vi "Day 7.1 - .vi"(11 "input":string[](array[string])) -> (1 "Sizes":i32[](array[numeric]), 2 "Dirs":string[](array[string]), 3 "output":u64)   [LabVIEW 2021]
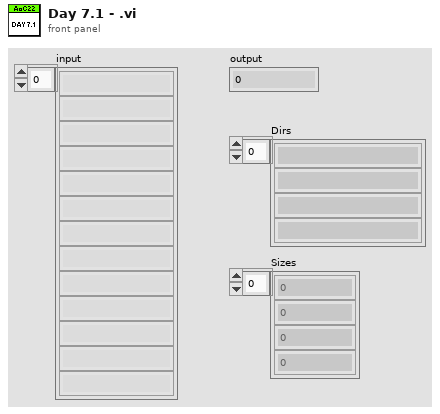
[diagram p1: front panel]
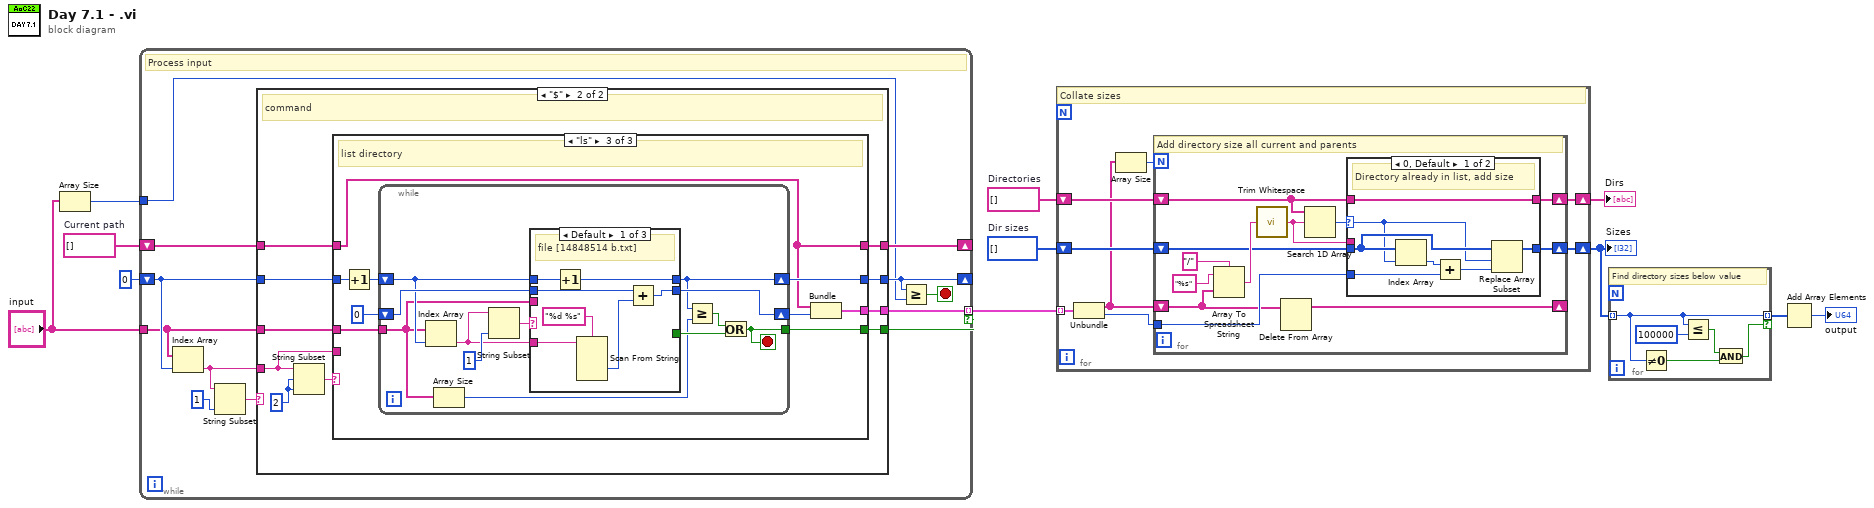
[diagram p0: block diagram]
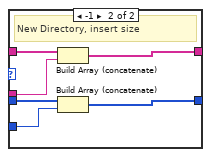
[diagram p2: hidden frame]
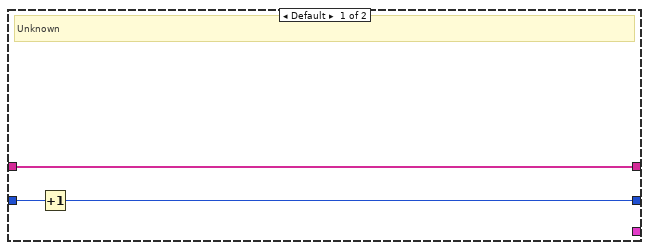
[diagram p3: hidden frame]
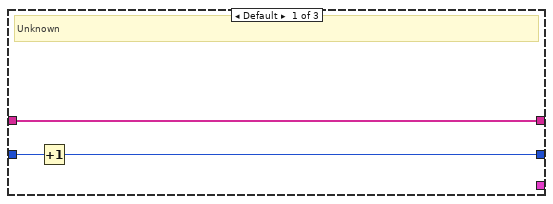
[diagram p4: hidden frame]
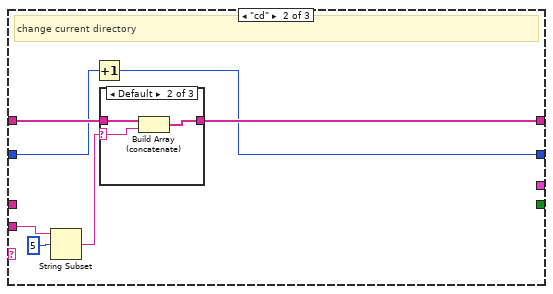
[diagram p5: hidden frame]
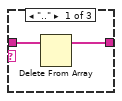
[diagram p6: hidden frame]
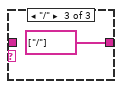
[diagram p7: hidden frame]
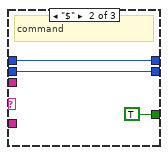
[diagram p8: hidden frame]
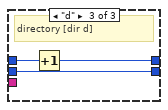
[diagram p9: hidden frame]
diagram:
  w3 = i32[] []  # Dir sizes
  w6 = string[] []  # Directories
  w10 = string[] []  # Current path
  n1 = Array Size(array="input") -> (size(s)=w8:i32)
  n2 = while {
    tunnel: "input" -> [w14]
    shift-right: [w17] -> _
    shift-left: i16 0 -> [w18]
    shift-right: [w20] -> _
    shift-left: w10 -> [w21]
    tunnel: w8 -> [w16]
    tunnel: [w13] -> w4 mode=indexing if=w12
    stop <- w15 stop-if-true
    # "Process input"
    n3 = Index Array(array=w14, index=w18) -> (element=w19:string)
    n4 = String Subset(string=w19, length (rest)=1 ("length (rest)")) -> (substring=w22:string)  [unwired: 1 in]
    n5 = case shown="\"$\"" w22 {
      tunnel: w19 -> [_ w35]
      tunnel: w21 -> [w26 w34]
      tunnel: [w26 w33] -> w20
      tunnel: w18 -> [w25 w32]
      tunnel: [w24 w31] -> w17
      tunnel: w14 -> [_ w30]
      tunnel: [_ w29] -> w13
      tunnel: [_ w28] -> w12
      frame Default {
        # "Unknown"
        n6 = Increment(x=w25) -> (x+1=w24:i16)
      }
      frame "$" {
        w27 = 2 ("length (rest)")
        # "command"
        n7 = String Subset(string=w35, offset (0)=w27, length (rest)=w27) -> (substring=w36:string)
        n8 = case shown="\"ls\"" w36 {
          tunnel: w35 -> [_ w46 _]
          tunnel: w34 -> [w39 w43 w53]
          tunnel: [w39 w42 w53] -> w33
          tunnel: w32 -> [w38 w41 w61]
          tunnel: [w37 w40 w58] -> w31
          tunnel: w30 -> [_ _ w60]
          tunnel: [_ _ w55] -> w29
          tunnel: [_ _ w54] -> w28
          frame Default {
            # "Unknown"
            n9 = Increment(x=w38) -> (x+1=w37:i16)
          }
          frame "cd" {
            # "change current directory"
            n10 = String Subset(string=w46, offset (0)=5) -> (substring=w44:string)  [unwired: 1 in]
            n11 = Increment(x=w41) -> (x+1=w40:i16)
            n12 = case shown="Default" w44 {
              selector: w44 -> [_ w50 _]
              tunnel: w43 -> [w48 w51 _]
              tunnel: [w47 w49 string[] ["/"]] -> w42
              frame ".." {
                n13 = Delete From Array(array=w48) -> (array with subset deleted=w47:string[])  [unwired: 2 in, 1 out]
              }
              frame Default {
                n14 = Build Array (concatenate)(w51, w50) -> (w49:string[])
              }
              frame "/" {
              }
            }
          }
          frame "ls" {
            # "list directory"
            n15 = Increment(x=w61) -> (x+1=w59:i16)
            n16 = while {
              tunnel: w60 -> [w65]
              shift-right: [w66] -> w58
              shift-left: w59 -> [w68]
              shift-right: [w70] -> w56
              shift-left: 0 -> [w71]
              tunnel: [w63] -> w54
              stop <- w63 stop-if-true
              n17 = Index Array(array=w65, index=w68) -> (element=w67:string)
              n18 = Array Size(array=w65) -> (size(s)=w64:i32)
              n19 = String Subset(string=w67, length (rest)=1 ("length (rest)")) -> (substring=w72:string)  [unwired: 1 in]
              n20 = case shown="Default" w72 {
                tunnel: w65 -> [_ _ _]
                tunnel: w68 -> [w80 w82 w86]
                tunnel: [w74 w82 w85] -> w66
                tunnel: [_ TRUE _] -> w69
                tunnel: w67 -> [w79 _ _]
                tunnel: w71 -> [w77 w81 w84]
                tunnel: [w75 w81 w84] -> w70
                frame Default {
                  # "file [14848514 b.txt]"
                  n21 = Increment(x=w80) -> (x+1=w74:i16)
                  n22 = Scan From String(format string="%d %s", input string=w79) -> (output 1=w76:i32)  [unwired: 5 in, 3 out]
                  n23 = Add(x=w77, y=w76) -> (x+y=w75:i32)
                }
                frame "$" {
                  # "command"
                }
                frame "d" {
                  # "directory [dir d]"
                  n24 = Increment(x=w86) -> (x+1=w85:i16)
                }
              }
              n25 = Greater Or Equal?(x=w66, y=w64) -> (x >= y?=w62:bool)
              n26 = Or(x=w62, y=w69) -> (x .or. y?=w63:bool)
            }
            n27 = Bundle("Current path"=w53, w56) -> (w55:cluster{"Current path":string[], i32})  [unwired: 1 in]
          }
        }
      }
    }
    n28 = Greater Or Equal?(x=w17, y=w16) -> (x >= y?=w15:bool)
  }
  n29 = for {
    tunnel: w4 -> [w94] mode=indexing
    shift-right: [w92] -> w5
    shift-left: w6 -> [w93]
    shift-right: [w89] -> w2
    shift-left: w3 -> [w91]
    # "Collate sizes"
    n30 = Unbundle(w94) -> ("Current path"=w88:string[], w90:i32)
    n31 = Array Size(array=w88) -> (size(s)=w87:i32)
    n32 = for {
      N: w87 -> [_]
      tunnel: w90 -> [w99]
      shift-right: [w101] -> w92
      shift-left: w93 -> [w102]
      shift-right: [w98] -> w89
      shift-left: w91 -> [w100]
      shift-right: [w96] -> _
      shift-left: w88 -> [w97]
      # "Add directory size all current and parents"
      n33 = Array To Spreadsheet String(delimiter (Tab)="/", array=w97, 3:"%s" ("format string")) -> (spreadsheet string=w103:string)
      n34 = call <vilib>:"Trim Whitespace.vi"("string"=w103) -> ("trimmed string"=w95:string)  [unwired: 1 in]
      n35 = Delete From Array(array=w97) -> (array with subset deleted=w96:string[])  [unwired: 2 in, 1 out]
      n36 = Search 1D Array(1D array=w102, element=w95) -> (index of element=w104:i32)  [unwired: 1 in]
      n37 = case shown="0, Default" w104 {
        selector: w104 -> [w109 _]
        tunnel: w95 -> [_ w118]
        tunnel: w102 -> [w113 w119]
        tunnel: [w113 w117] -> w101
        tunnel: w100 -> [w110 w116]
        tunnel: w99 -> [w107 w115]
        tunnel: [w111 w114] -> w98
        frame 0, Default {
          # "Directory already in list, add size"
          n38 = Index Array(array=w110, index=w109) -> (element=w112:i32)
          n39 = Add(x=w112, y=w107) -> (x+y=w108:i32)
          n40 = Replace Array Subset(array=w110, new element=w108, index=w109) -> (w111:i32[])
        }
        frame -1 {
          # "New Directory, insert size"
          n41 = Build Array (concatenate)(w119, w118) -> (w117:string[])
          n42 = Build Array (concatenate)(w116, w115) -> (w114:i32[])
        }
      }
    }
  }
  "Dirs" <- w5
  "Sizes" <- w2
  n43 = for {
    tunnel: w2 -> [w120] mode=indexing
    tunnel: [w120] -> w1 mode=indexing if=w121
    # "Find directory sizes below value"
    n44 = Not Equal To 0?(x=w120) -> (x != 0?=w124:bool)
    n45 = Less Or Equal?(x=w120, y=100000) -> (x <= y?=w123:bool)
    n46 = And(x=w123, y=w124) -> (x .and. y?=w121:bool)
  }
  n47 = Add Array Elements(numeric array=w1) -> (sum=→"output":i32)
